vi "Name Request.vi"(8 "error in (no error)":errorcluster, 11 "BuildWorker in":refnum<class "BuildWorker.lvclass">) -> (0 "error out":errorcluster, 3 "BuildWorker out":refnum<class "BuildWorker.lvclass">)   [LabVIEW 2017, in "BuildWorker.lvlib" / "BuildWorker.lvclass"]
uses:
  BuildWorker.lvclass
  BuildWorker.lvclass/BuildWorker.ctl
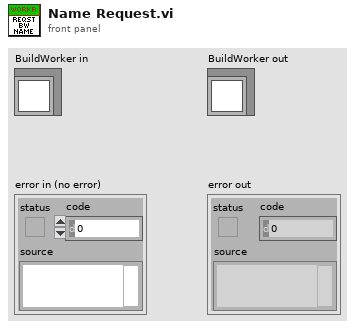
[diagram p1: front panel]
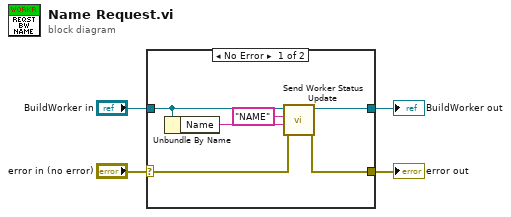
[diagram p0: block diagram]
diagram:
  n1 = case shown="No Error" "error in (no error)" {
    selector: "error in (no error)" -> [w6 w12]
    tunnel: [w5 w12] -> w1
    tunnel: [w9 w11] -> w2
    tunnel: "BuildWorker in" -> [w10 w11]
    frame No Error {
      n2 = Unbundle By Name(w10) -> ("Name"=w8:string)
      n3 = call "Send Worker Status Update.vi"("error in (no error)"=w6, "Status"=w8, "Operation"="NAME", "BuildWorker in"=w10) -> ("error out"=w5:errorcluster, "BuildWorker out"=w9:refnum<class "BuildWorker.lvclass">)  [unwired: 6 in]
    }
    frame Error {
    }
  }
  "error out" <- w1
  "BuildWorker out" <- w2
